vi "test_Bitfile Reload_Scalar Data Type Change FXP.vi"(8 "error in (no error)":errorcluster, 11 "TestCase in":refnum<class "Bitfile Reload System Tests.lvclass">) -> (0 "error out":errorcluster, 3 "TestCase out":refnum<class "Bitfile Reload System Tests.lvclass">)   [LabVIEW 2021, in "Bitfile Reload System Tests.lvclass"]
uses:
  Bitfile Reload System Tests.lvclass
  C:/Program Files/National Instruments/LabVIEW 2021/vi.lib/NI/VeriStand Custom Device Testing Tools/VeriStandTestCase/VeriStandTestCase.lvclass
  APIs/Scripting API/TypeDefs/Output Scalar Data.ctl
  Addon/Addon Shared/Types/FPGA Addon Data Type.ctl
  <vilib>/NI VeriStand/Execution/Workspace/NI VeriStand - Get Single Channel Value.vi
  <vilib>/addons/_JKI Toolkits/VI Tester/TestCase.llb/TestCase.lvclass
  FPGA Addon Test Class/FPGA Addon Test Class.lvclass
  Addon/Addon System Explorer/FPGA Addon System Explorer.lvlib
  APIs/Scripting API/Scripting API.lvlib
  <vilib>/NI VeriStand/Execution/Workspace/NI_VS Workspace ExecutionAPI.lvlib
  Addon/Addon Shared/FPGA Addon Shared.lvlib
  C:/Program Files/National Instruments/LabVIEW 2021/vi.lib/addons/_JKI Toolkits/VI Tester/TestCase.llb/TestCase.lvclass
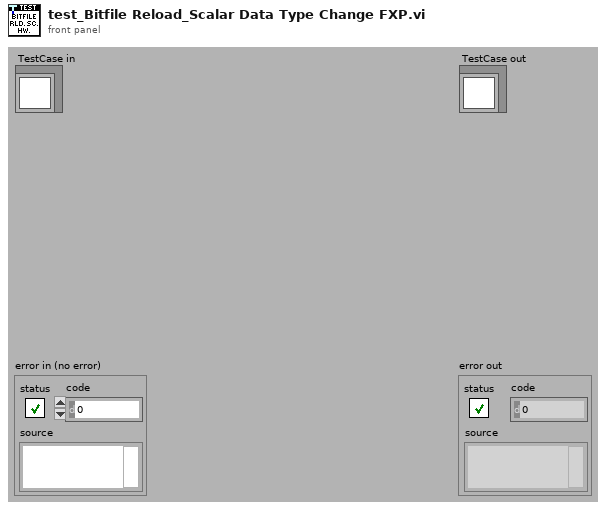
[diagram p1: front panel]
types:
  T1 = typedef "Scripting API.lvlib/Output Scalar Data.ctl" = cluster{"Bitfile Name":string, "SysDef Channel Name":string, "Imported":bool, "Data Type":T2}
  T2 = typedef "FPGA Addon Shared.lvlib/FPGA Addon Data Type.ctl" = enum8{"<Null>", "I8", "I16", "I32", "I64", "U8", "U16", "U32", "U64", "SGL", "Boolean", "Analog PWM In Settings", "Analog PWM In", "Digital PWM In Settings", "Digital PWM In", "Digital PWM Out", "Sine Out", "FXP", "FXP+/-24.5", "FXP+/-16.5", "FXP+/-32.8", "FXP+/-64.32", "FXP+/-16.7", "FXP+/-20.5", "FXP+/-27.5", "FXP+/-32.16", "FXP+16.3", "FXP+18.3", "Digital Static In", "Digital Static Out", "Digital Static In Settings", "Digital WSS Out", "Quad Encoder Settings", "Quad Encoder In", "Group"}
  T3 = typedef "Custom Device API.lvlib/Custom Device Item Ref.ctl" = u64
  T4 = typedef "NI_VS Workspace ExecutionAPI.lvlib/WorkspaceAPI.ctl" = refnum<k24>
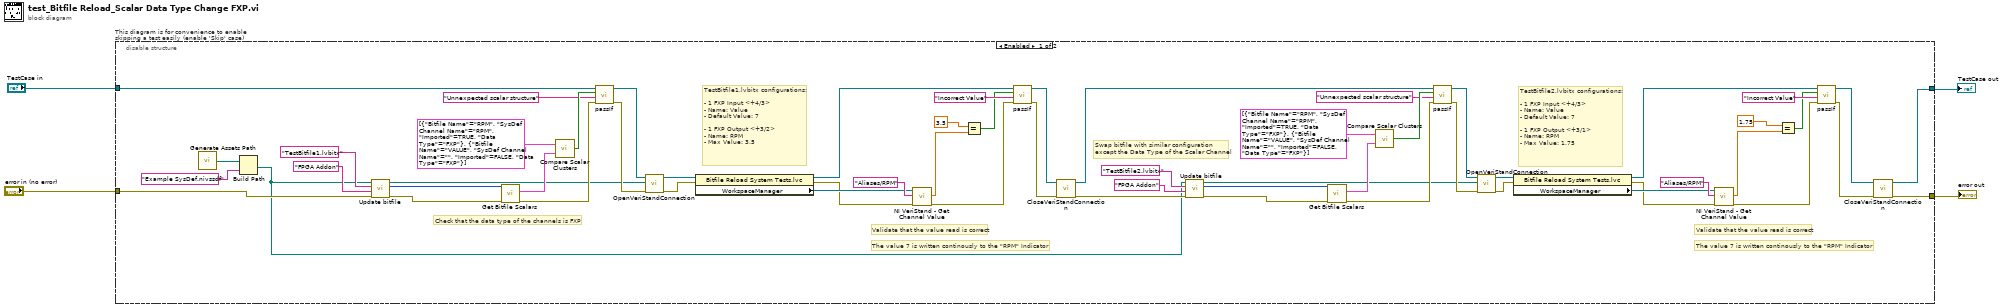
[diagram p0: block diagram]
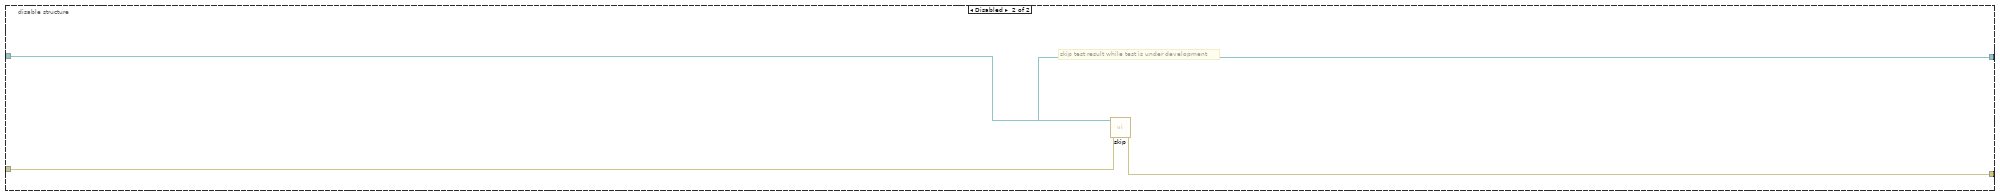
[diagram p2: hidden frame]
diagram:
  n1 = disable-structure "This diagram is for convenience to enable skipping a test easily (enable 'Skip' case)" shown="Enabled" {
    disable-tunnel: "TestCase in" -> [w58 w67]
    disable-tunnel: [w24 w65] -> w1
    disable-tunnel: [w20 w66] -> w3
    disable-tunnel: "error in (no error)" -> [w19 w64]
    frame Enabled {
      # "The value 7 is written continously to the \"RPM\" Indicator"
      # "The value 7 is written continously to the \"RPM\" Indicator"
      # "Validate that the value read is correct"
      # "Swap bitfile with similar configuration\nexcept the Data Type of the Scalar Channel"
      # "Validate that the value read is correct"
      # "TestBitfile2.lvbitx configurations:\n\n- 1 FXP Input <+4/3>\n- Name: Value\n- Default Value: 7\n\n- 1 FXP Output <+3/1>\n- Name: RPM\n- Max Value: 1.75"
      # "TestBitfile1.lvbitx configurations:\n\n- 1 FXP Input <+4/3>\n- Name: Value\n- Default Value: 7\n\n- 1 FXP Output <+3/2>\n- Name: RPM\n- Max Value: 3.5"
      # "Check that the data type of the channels is FXP"
      n2 = call "Generate Assets Path.vi"() -> ("Assets path"=w62:path)
      n3 = Build Path(base path=w62, name or relative path="Example SysDef.nivssdf") -> (appended path=w11:path)
      n4 = call "Update bitfile.vi"("error in (no error)"=w19, "FPGA addon name"="FPGA Addon", "bitfile name"="TestBitfile1.lvbitx", "sysdef path in"=w11) -> ("error out"=w18:errorcluster, "FPGA addon refnum out"=w15:T3, "sysdef path out"=w12:path)  [unwired: 5 in]
      n5 = call "Get Bitfile Scalars.vi"("error in"=w18, "FPGA addon refnum in"=w15) -> ("error out"=w57:errorcluster, "bitfile scalars out"=w60:T1[])  [unwired: 7 in, 1 out]
      n6 = call "Compare Scalar Clusters.vi"("Target bitfile scalars in"=w60, "Reference bitfile scalars in"=T1[] [{"Bitfile Name"="RPM", "SysDef Channel Name"="RPM", "Imported"=TRUE, "Data Type"=enum."FXP"}, {"Bitfile Name"="VALUE", "SysDef Channel Name"="", "Imported"=FALSE, "Data Type"=enum."FXP"}] ("bitfile scalars out")) -> ("Equal ?"=w56:bool)
      n7 = call-dynamic "passIf.vi"("error in (no error)"=w57, "message (\"\")"="Unnexpected scalar structure" ("message (\"\")"), "pass"=w56, "TestCase in"=w58) -> ("error out"=w54:errorcluster, "TestCase out"=w59:refnum<class "Bitfile Reload System Tests.lvclass">)  [unwired: 6 in]
      n8 = call-dynamic "OpenVeriStandConnection.vi"("error in (no error)"=w54, "System Definition File"=w12, "VeriStand Test Case in"=w59) -> ("error out"=w31:errorcluster, "VeriStand Test Case out"=w32:refnum<class "Bitfile Reload System Tests.lvclass">)  [unwired: 6 in, 1 out]
      n9 = property class="Bitfile Reload System Tests.lvc"(reference=w32, error in=w31) -> (reference out=w48:refnum<class "Bitfile Reload System Tests.lvclass">, error out=w45:errorcluster, "WorkspaceManager"=w46:T4)
      n10 = call-poly <vilib>:"NI VeriStand - Get Channel Value.vi"("error in (no error)"=w45, "Channel"="Aliases/RPM", "WorkspaceManager in"=w46) -> ("error out"=w9:errorcluster, "Value"=w23:dbl)  [unwired: 6 in, 1 out]
      n11 = Equal?(x=3.5, y=w23) -> (x = y?=w21:bool)
      n12 = call-dynamic "passIf.vi"("error in (no error)"=w9, "message (\"\")"="Incorrect Value" ("message (\"\")"), "pass"=w21, "TestCase in"=w48) -> ("error out"=w50:errorcluster, "TestCase out"=w51:refnum<class "Bitfile Reload System Tests.lvclass">)  [unwired: 6 in]
      n13 = call-dynamic "CloseVeriStandConnection.vi"("error in (no error)"=w50, "VeriStand Test Case in"=w51) -> ("error out"=w44:errorcluster, "VeriStand Test Case out"=w40:refnum<class "Bitfile Reload System Tests.lvclass">)  [unwired: 8 in]
      n14 = call "Update bitfile.vi"("error in (no error)"=w44, "FPGA addon name"="FPGA Addon", "bitfile name"="TestBitfile2.lvbitx", "sysdef path in"=w11) -> ("error out"=w14:errorcluster, "FPGA addon refnum out"=w13:T3, "sysdef path out"=w10:path)  [unwired: 5 in]
      n15 = call "Get Bitfile Scalars.vi"("error in"=w14, "FPGA addon refnum in"=w13) -> ("error out"=w35:errorcluster, "bitfile scalars out"=w37:T1[])  [unwired: 7 in, 1 out]
      n16 = call "Compare Scalar Clusters.vi"("Target bitfile scalars in"=w37, "Reference bitfile scalars in"=T1[] [{"Bitfile Name"="RPM", "SysDef Channel Name"="RPM", "Imported"=TRUE, "Data Type"=enum."FXP"}, {"Bitfile Name"="VALUE", "SysDef Channel Name"="", "Imported"=FALSE, "Data Type"=enum."FXP"}] ("bitfile scalars out")) -> ("Equal ?"=w34:bool)
      n17 = call-dynamic "passIf.vi"("error in (no error)"=w35, "message (\"\")"="Unnexpected scalar structure" ("message (\"\")"), "pass"=w34, "TestCase in"=w40) -> ("error out"=w38:errorcluster, "TestCase out"=w39:refnum<class "Bitfile Reload System Tests.lvclass">)  [unwired: 6 in]
      n18 = call-dynamic "OpenVeriStandConnection.vi"("error in (no error)"=w38, "System Definition File"=w10, "VeriStand Test Case in"=w39) -> ("error out"=w29:errorcluster, "VeriStand Test Case out"=w30:refnum<class "Bitfile Reload System Tests.lvclass">)  [unwired: 6 in, 1 out]
      n19 = property class="Bitfile Reload System Tests.lvc"(reference=w30, error in=w29) -> (reference out=w26:refnum<class "Bitfile Reload System Tests.lvclass">, error out=w27:errorcluster, "WorkspaceManager"=w28:T4)
      n20 = call-poly <vilib>:"NI VeriStand - Get Channel Value.vi"("error in (no error)"=w27, "Channel"="Aliases/RPM", "WorkspaceManager in"=w28) -> ("error out"=w42:errorcluster, "Value"=w5:dbl)  [unwired: 6 in, 1 out]
      n21 = Equal?(x=1.75, y=w5) -> (x = y?=w6:bool)
      n22 = call-dynamic "passIf.vi"("error in (no error)"=w42, "message (\"\")"="Incorrect Value" ("message (\"\")"), "pass"=w6, "TestCase in"=w26) -> ("error out"=w8:errorcluster, "TestCase out"=w25:refnum<class "Bitfile Reload System Tests.lvclass">)  [unwired: 6 in]
      n23 = call-dynamic "CloseVeriStandConnection.vi"("error in (no error)"=w8, "VeriStand Test Case in"=w25) -> ("error out"=w20:errorcluster, "VeriStand Test Case out"=w24:refnum<class "Bitfile Reload System Tests.lvclass">)  [unwired: 8 in]
      n24 = call "Reload Bitfile.vi"() -> ()  [unwired: 10 in, 2 out]
    }
    frame Disabled {
      # "skip test result while test is under development"
      n25 = call <vilib>:"skip.vi"("error in (no error)"=w64, "TestCase in"=w67) -> ("error out"=w66:errorcluster, "TestCase out"=w65:refnum<class "Bitfile Reload System Tests.lvclass">)  [unwired: 8 in]
    }
  }
  "error out" <- w3
  "TestCase out" <- w1
